vi "Grafica_XY.vi"() -> ()   [LabVIEW 2016]
panel:
  out "XY Graph":cluster{dbl[], dbl[]}(graph)
  out "Waveform Graph 2":dbl[](graph)
  out "Waveform Graph":dbl[](graph)
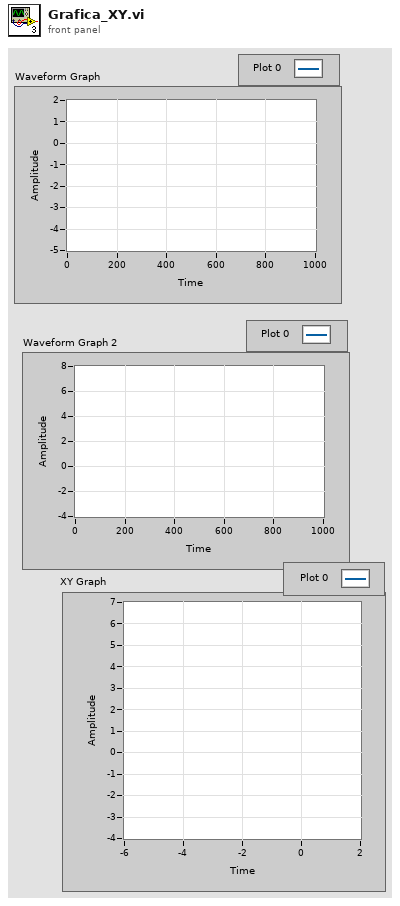
[diagram p1: front panel]
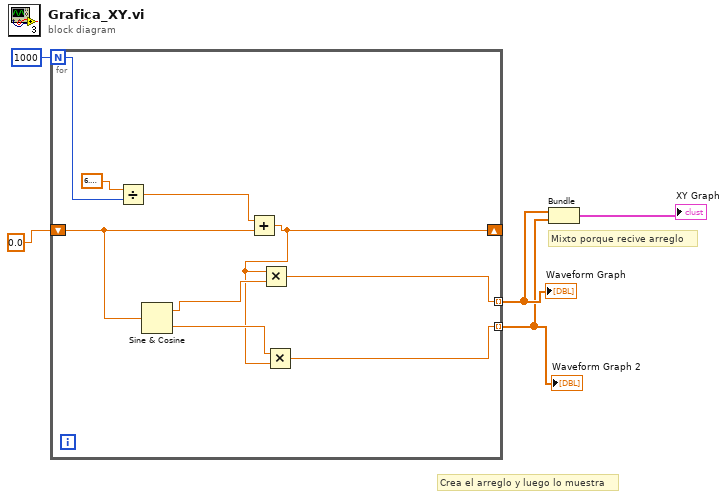
[diagram p0: block diagram]
diagram:
  # "Mixto porque recive arreglo"
  # "Crea el arreglo y luego lo muestra"
  n1 = for {
    N: 1000 -> [w13]
    shift-right: [w6] -> _
    shift-left: 0.0 -> [w11]
    tunnel: [w7] -> w3 mode=indexing
    tunnel: [w8] -> w2 mode=indexing
    n2 = Divide(x=6.283185307179586, y=w13) -> (x/y=w12:dbl)
    n3 = Sine & Cosine(0:w11) -> (1:w10:dbl, 2:w9:dbl)
    n4 = Add(x=w12, y=w11) -> (x+y=w6:dbl)
    n5 = Multiply(x=w6, y=w10) -> (x*y=w7:dbl)
    n6 = Multiply(x=w9, y=w6) -> (x*y=w8:dbl)
  }
  "Waveform Graph 2" <- w2
  "Waveform Graph" <- w3
  n7 = Bundle(w3, w2) -> (→"XY Graph":cluster{dbl[], dbl[]})  [unwired: 1 in]
